vi "GOOP_GetClassWriterByClassRef.vi"(1 "LVClassLibrary Refnum":refnum<vi>, 5 "error in (no error)":errorcluster) -> (14 "ClassWriterNative.lvclass":refnum<class "ClassWriterNative.lvclass">, 19 "error out":errorcluster)   [LabVIEW 2020]
uses:
  <resource>/Framework/Providers/Open_GDS/ClassProviders/Provider_LvNativeClass/ClassWriterNative_class/ClassWriterNative.lvclass
  <resource>/Framework/Providers/Open_GDS/ClassProviders/Provider_LvNativeClass/LvNativeProviderName.ctl
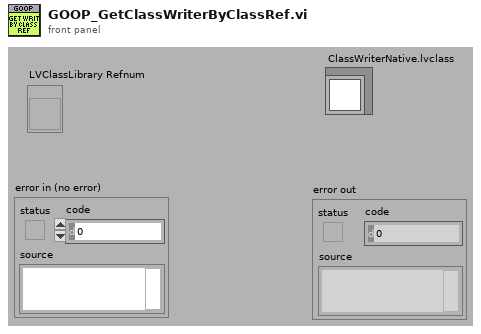
[diagram p1: front panel]
types:
  T1 = typedef "LvNativeProviderName.ctl" = enum16{"Endevo LabVIEW Native"}
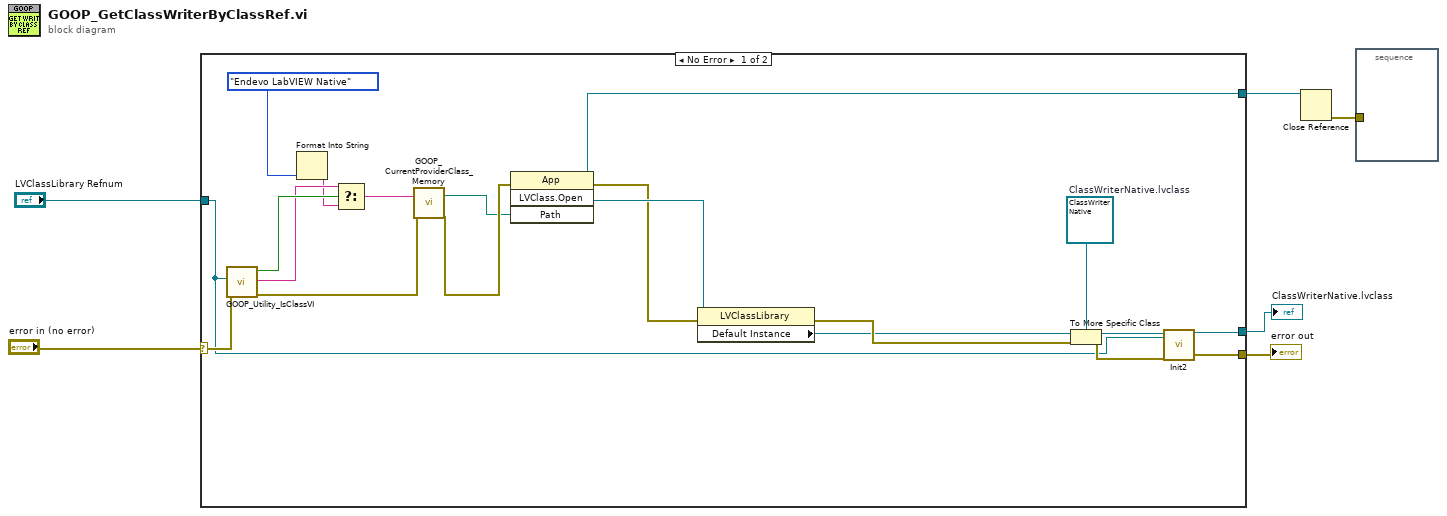
[diagram p0: block diagram]
diagram:
  n1 = case shown="No Error" "error in (no error)" {
    selector: "error in (no error)" -> [w26 w27]
    tunnel: "LVClassLibrary Refnum" -> [w7 _]
    tunnel: [w15 w27] -> w4
    tunnel: [w16 _] -> w2
    tunnel: [w13 _] -> w3
    frame No Error {
      w8 = refnum<class "ClassWriterNative.lvclass"> refnum  # ClassWriterNative.lvclass
      n2 = call <resource>:"GOOP_Utility_IsClassVI.vi"("error in (no error)"=w26, "ProjectItem"=w7) -> ("error out"=w25:errorcluster, "ClassProvider"=w23:string, "Is Class VI?"=w24:bool)  [unwired: 4 in, 3 out]
      n3 = Format Into String(LvNativeProviderName."Endevo LabVIEW Native" ("ProviderName")) -> (resulting string=w20:string)  [unwired: 3 in, 1 out]
      n4 = Select(t=w23, s=w24, f=w20) -> (s? t:f=w22:string)
      n5 = call <resource>:"GOOP_CurrentProviderClass_Memory.vi"("GetThisClassProvidersPaths(Returns the default providor if not wired)"=w22, "error in (no error)"=w25) -> ("ClassProviderClassWriterPath"=w9:path, "error out"=w19:errorcluster)  [unwired: 11 in, 5 out]
      n6 = invoke class="App" method="LVClass.Open"(error in=w19, "Path"=w9) -> (reference out=w13:refnum<vi>, error out=w12:errorcluster, "LVClass.Open"=w18:refnum<vi>)  [unwired: 2 in, 1 out]
      n7 = property class="LVClassLibrary"(reference=w18, error in=w12) -> (error out=w11:errorcluster, "Default Instance"=w10:refnum<class>)  [unwired: 1 out]
      n8 = To More Specific Class(target class=w8, reference=w10, error in=w11) -> (specific class reference=w14:refnum<class "ClassWriterNative.lvclass">, error out=w17:errorcluster)
      n9 = call-dynamic "Init2.vi"("ClassWriterNative.lvclass"=w14, "LvClassRef"=w7, "error in (no error)"=w17) -> ("ClassWriterNative.lvclass"=w16:refnum<class "ClassWriterNative.lvclass">, "error out"=w15:errorcluster)  [unwired: 15 in]
    }
    frame Error {
    }
  }
  "error out" <- w4
  "ClassWriterNative.lvclass" <- w2
  n10 = Close Reference(reference=w3) -> (error out=w1:errorcluster)  [unwired: 1 in]
  n11 = stacked-sequence {
    tunnel: w1 -> [_]
    frame #0 {
    }
  }
